vi "navXPacketParser.vi"(4 "Message":u8[](array[numeric])) -> (1 "navXPacket":T1)   [LabVIEW 2014]
uses:
  navXPacket.ctl
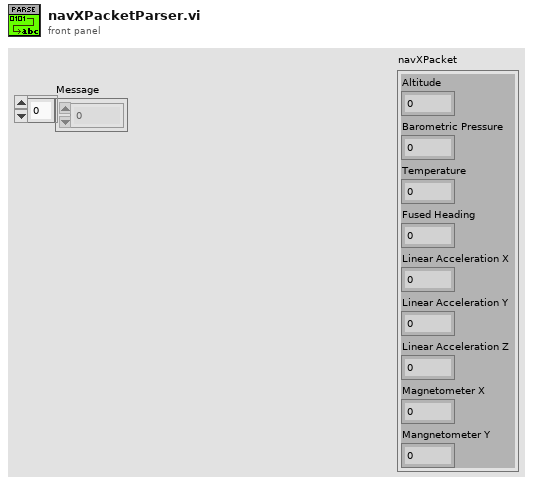
[diagram p1: front panel]
types:
  T1 = typedef "navXPacket.ctl" = cluster{"Altitude":dbl, "Barometric Pressure":dbl, "Fused Heading":dbl, "Linear Acceleration Y":dbl, "Linear Acceleration X":dbl, "Temperature":dbl, "Mangnetometer Y":dbl, "Magnetometer X":dbl, "Linear Acceleration Z":dbl}
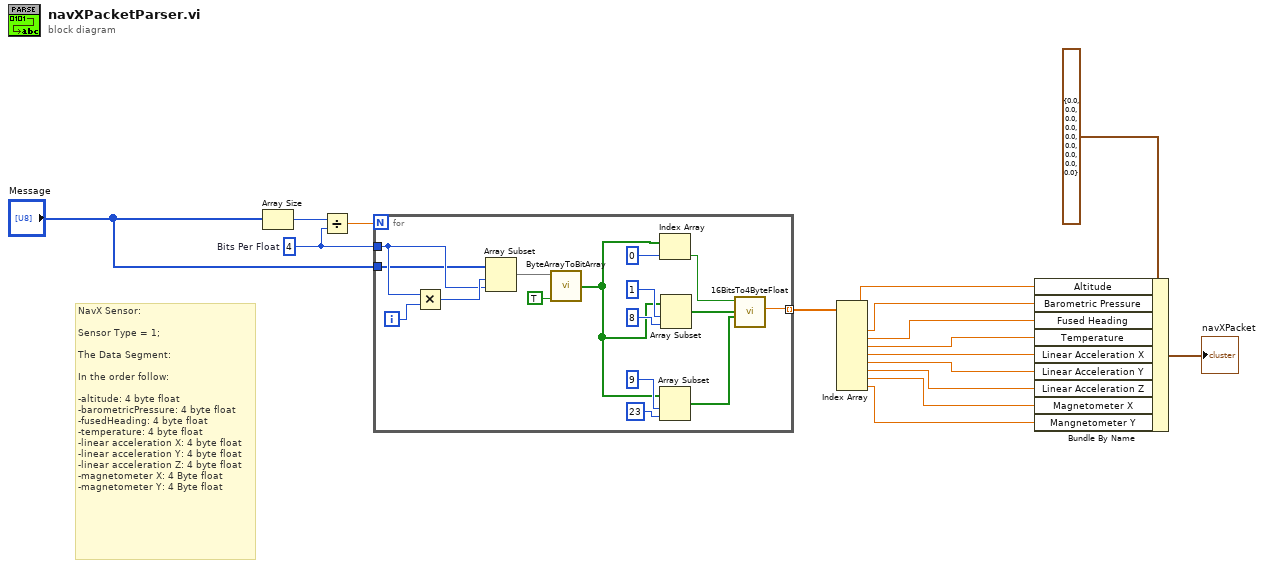
[diagram p0: block diagram]
diagram:
  w14 = 4  # Bits Per Float
  # "NavX Sensor:\n\nSensor Type = 1;\n\nThe Data Segment:\n\nIn the order follow:\n\n-altitude: 4 byte float\n-barometricPressure: 4 byte float\n-fusedHeading: 4 byte float\n-temperature: 4 byte float\n-linear acceleration X: 4 byte float\n-linear acceleration Y: 4 byte float\n-linear acceleration Z: 4 byte float\n-magnetometer X: 4 Byte float\n-magnetometer Y: 4 Byte float"
  n1 = Array Size(array="Message") -> (size(s)=w16:i32)
  n2 = Divide(x=w16, y=w14) -> (x/y=w15:dbl)
  n3 = for {
    N: w15 -> [_]
    tunnel: w14 -> [w30]
    tunnel: "Message" -> [w29]
    tunnel: [w28] -> w13 mode=indexing
    i -> [w32]
    n4 = Multiply(x=w30, y=w32) -> (x*y=w31:i32)
    n5 = Array Subset(array=w29, index=w31, length=w30) -> (w19:u8[])
    n6 = call "ByteArrayToBitArray.vi"("Flip Endian"=TRUE, "Byte Array In"=w19) -> ("Bit Array Out"=w17:bool[])  [unwired: 4 in]
    n7 = Index Array(array=w17, index=0) -> (element=w20:bool)
    n8 = Array Subset(array=w17, index=9, length=23) -> (w24:bool[])
    n9 = Array Subset(array=w17, index=1, length=8) -> (w27:bool[])
    n10 = call "16BitsTo4ByteFloat.vi"("Array"=w24, "Array 2"=w27, "Sign"=w20) -> ("Numeric"=w28:sgl)  [unwired: 6 in, 2 out]
  }
  n11 = Index Array(array=w13) -> (element #1=w11:sgl, element #2=w10:sgl, element #3=w9:sgl, element #4=w8:sgl, element #5=w7:sgl, element #6=w6:sgl, element #7=w5:sgl, element #8=w4:sgl, element #9=w3:sgl)  [unwired: 9 in]
  n12 = Bundle By Name(cluster=T1 {"Altitude"=0.0, "Barometric Pressure"=0.0, "Fused Heading"=0.0, "Linear Acceleration Y"=0.0, "Linear Acceleration X"=0.0, "Temperature"=0.0, "Mangnetometer Y"=0.0, "Magnetometer X"=0.0, "Linear Acceleration Z"=0.0} ("navXPacket 2"), "Altitude"=w11, "Barometric Pressure"=w10, "Fused Heading"=w9, "Temperature"=w8, "Linear Acceleration X"=w7, "Linear Acceleration Y"=w6, "Linear Acceleration Z"=w5, "Magnetometer X"=w4, "Mangnetometer Y"=w3) -> (→"navXPacket":T1)
